vi "ESP Read-Write (SubVI) - C.vi"(0 "COM Port Input":refnum<visa-resource-name>, 5 "Command Input":T2, 7 "Manual Write Command":bool, 9 "Timeout (ms)":u32=10, 11 "Write/Read Wait (ms)":u32=10, 12 "Auto-Write on New Command?":bool=TRUE, 14 "Stop Program?":bool) -> (4 "ESP Values":T1, 15 "Error Output":errorcluster)   [LabVIEW 2011]
panel:
  # "ESP-D Read/Write (SubVI)\nCreated by Blake Otting - November 2009\nLast Updated - 2-29-2012"
  # "OUTPUTS"
  # "INPUTS"
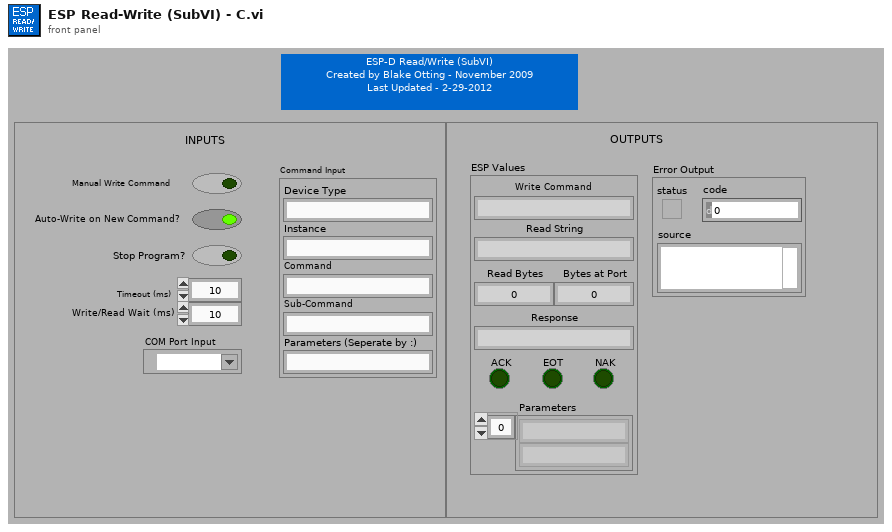
[diagram p1: front panel]
types:
  T1 = cluster{"Write Command":string, "Read String":string, "Read Bytes":u32, "Bytes at Port":u32, "Response":string, "ACK":bool, "EOT":bool, "NAK":bool, "Parameters":string[]}
  T2 = cluster{"Device Type":string, "Instance":string, "Command":string, "Sub-Command":string, "Parameters (Seperate by :)":string}
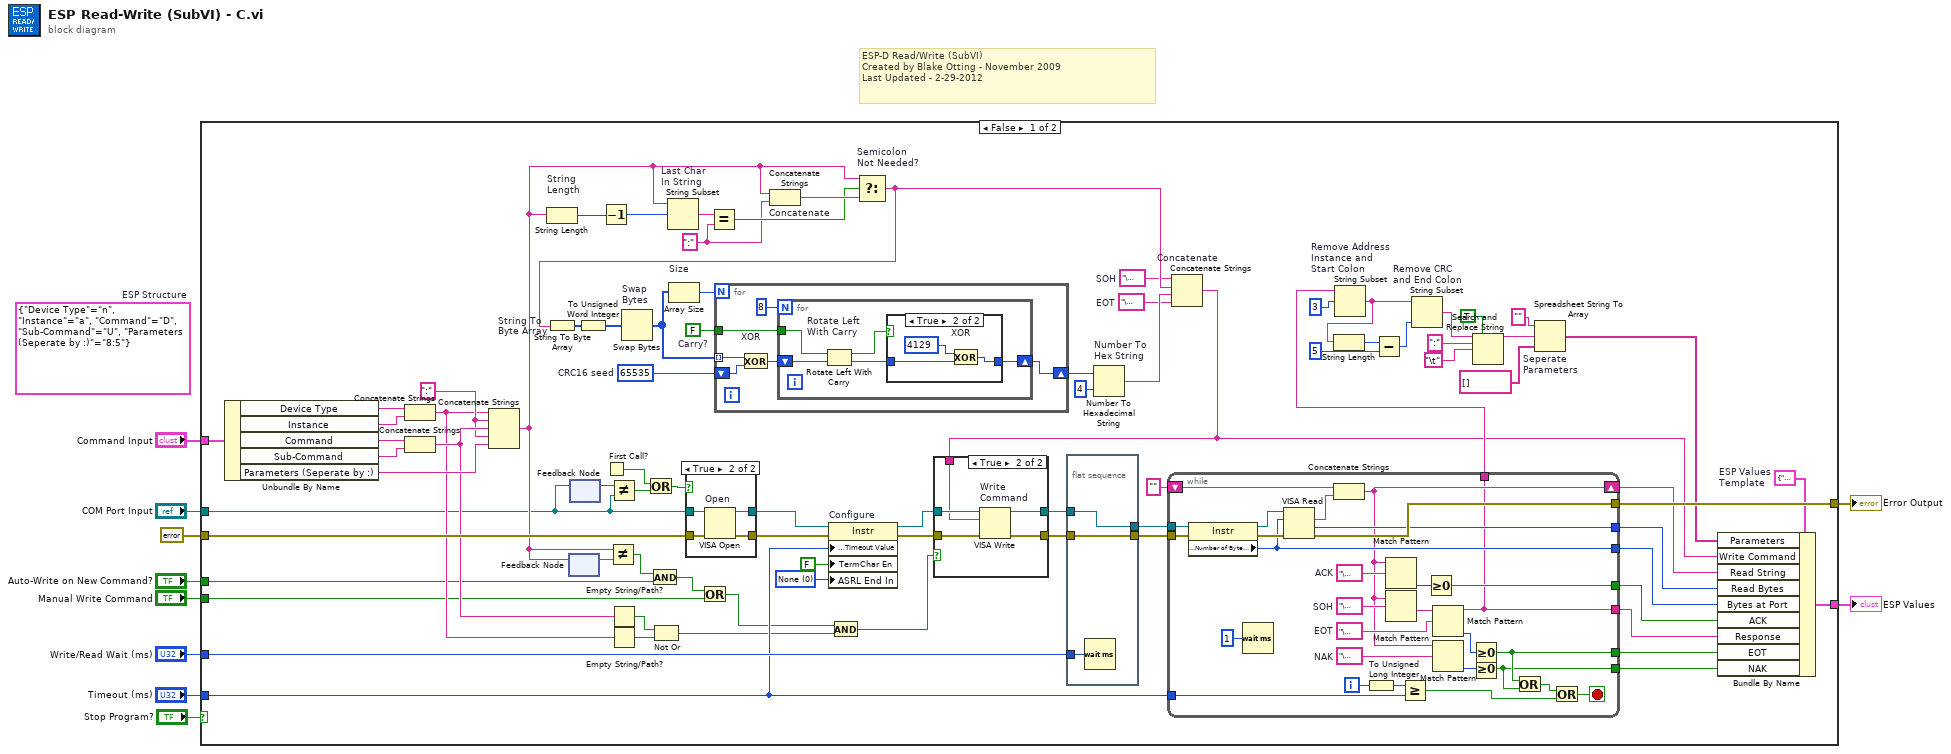
[diagram p0: block diagram]
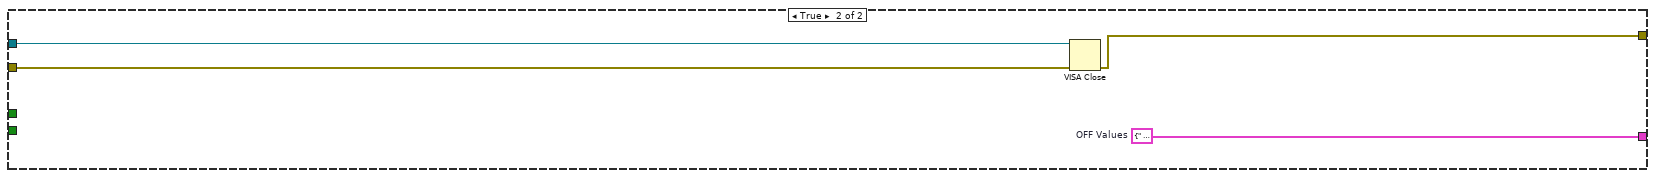
[diagram p5: hidden frame]
diagram:
  (unwired) T2 {"Device Type"="n", "Instance"="a", "Command"="D", "Sub-Command"="U", "Parameters (Seperate by :)"="8:5"}  # ESP Structure
  # "ESP-D Read/Write (SubVI)\nCreated by Blake Otting - November 2009\nLast Updated - 2-29-2012"
  n1 = case shown="False" "Stop Program?" {
    tunnel: "Auto-Write on New Command?" -> [w19 _]
    tunnel: "Command Input" -> [w92 _]
    tunnel: "Manual Write Command" -> [w18 _]
    tunnel: "Timeout (ms)" -> [w48 _]
    tunnel: "Write/Read Wait (ms)" -> [w91 _]
    tunnel: [w47 w154] -> w5
    tunnel: "COM Port Input" -> [w21 w156]
    tunnel: [w73 w153] -> w1
    tunnel: errorcluster {"status"=FALSE, "code"=0, "source"=""} ("error in (no error)") -> [w68 w155]
    frame False {
      w11 = FALSE  # Carry?
      w42 = T1 {"Write Command"="", "Read String"="", "Read Bytes"=0, "Bytes at Port"=0, "Response"="", "ACK"=FALSE, "EOT"=FALSE, "NAK"=FALSE, "Parameters"=[]}  # ESP Values  Template
      w49 = "\u0004"  # EOT
      w50 = "\u0001"  # SOH
      w85 = ":" ("y")
      w77 = u16 65535  # CRC16 seed
      w66 = u16 0 items=["None", "LastBit", "TermChar"] ("ASRLEndIn")
      w28 = ":"
      n2 = Unbundle By Name(w92) -> ("Device Type"=w34:string, "Instance"=w33:string, "Command"=w32:string, "Sub-Command"=w31:string, "Parameters (Seperate by :)"=w30:string)
      n3 = Concatenate Strings(w34, w33) -> (w27:string)
      n4 = Concatenate Strings(w32, w31) -> (w29:string)
      n5 = Concatenate Strings(w27, w28, w29, w28, w30) -> (w24:string)
      n6 = String Length "String\nLength"(string=w24) -> (length=w82:i32)
      n7 = feedback-in #1(w24) -> ()
      n8 = feedback #1() -> (w23:string)  [unwired: 1 in]
      n9 = feedback #2() -> (w22:refnum<visa-resource-name>)  [unwired: 1 in]
      n10 = feedback-in #2(w21) -> ()
      n11 = Decrement(x=w82) -> (x-1=w83:i32)
      n12 = First Call?() -> (First Call?: T/F=w13:bool)
      n13 = Not Equal?(x=w24, y=w23) -> (x != y?=w20:bool)
      n14 = Not Equal?(x=w22, y=w21) -> (x != y?=w12:bool)
      n15 = Empty String/Path?(string/path=w29) -> (empty?=w26:bool)
      n16 = Empty String/Path?(string/path=w27) -> (empty?=w25:bool)
      n17 = Or(x=w13, y=w12) -> (x .or. y?=w74:bool)
      n18 = And(x=w20, y=w19) -> (x .and. y?=w17:bool)
      n19 = Not Or(1:w25, 2:w26) -> (0:w15:bool)
      n20 = String Subset "Last Char\nIn String"(string=w24, offset (0)=w83) -> (substring=w84:string)  [unwired: 1 out]
      n21 = case shown="True" w74 {
        tunnel: w21 -> [w123 w127]
        tunnel: [w123 w126] -> w72
        tunnel: w68 -> [w122 w125]
        tunnel: [w122 w124] -> w71
        frame False {
        }
        frame True {
          n22 = VISA Open "Open"(error in (no error)=w125, VISA resource name=w127) -> (VISA resource name=w126:refnum<visa-resource-name>, error out=w124:errorcluster)  [unwired: 3 in]
        }
      }
      n23 = Or(x=w17, y=w18) -> (x .or. y?=w16:bool)
      n24 = Equal?(x=w84, y=w85) -> (x = y?=w86:bool)
      n25 = Concatenate Strings "Concatenate"(w24, w85) -> (w87:string)
      n26 = property on="Configure" class="Instr"(reference=w72, error in=w71, "General Settings:Timeout Value"=w48, "TermChar En"=FALSE ("enable"), "ASRL End In"=w66) -> (reference out=w70:refnum<visa-resource-name>, error out=w69:errorcluster)
      n27 = And(x=w16, y=w15) -> (x .and. y?=w14:bool)
      n28 = Select "Semicolon\nNot Needed?"(t=w24, s=w86, f=w87) -> (s? t:f=w88:string)
      n29 = String To Byte Array "String To \nByte Array"(string=w88) -> (unsigned byte array=w75:u8[])
      n30 = To Unsigned Word Integer ("To\nUNIT16")(number=w75) -> (unsigned 16bit integer=w76:u16[])
      n31 = Swap Bytes "Swap\nBytes"(anything=w76) -> (byte swapped=w79:u16[])
      n32 = Array Size "Size"(array=w79) -> (size(s)=w78:i32)
      n33 = for {
        N: w78 -> [_]
        shift-right: [w132] -> w80
        shift-left: w77 -> [w129]
        tunnel: w79 -> [w131] mode=indexing
        tunnel: w11 -> [w128]
        n34 = Exclusive Or "XOR"(1:w129, 2:w131) -> (0:w130:u16)
        n35 = for {
          N: 8 -> [_]
          shift-right: [w138] -> w132
          shift-left: w130 -> [w135]
          tunnel: w128 -> [w134]
          n36 = Rotate Left With Carry "Rotate Left\nWith Carry"(2:w135, 3:w134) -> (0:w136:u16, 1:w137:bool)
          n37 = case shown="True" w137 {
            tunnel: w136 -> [w139 w140]
            tunnel: [w139 w142] -> w138
            frame False {
            }
            frame True {
              n38 = Exclusive Or "XOR"(1:w140, 2:u16 4129) -> (0:w142:u16)
            }
          }
        }
      }
      n39 = flat-sequence {
        tunnel: w89 -> [w145]
        tunnel: [w145] -> w51
        tunnel: w90 -> [w144]
        tunnel: [w144] -> w52
        tunnel: w91 -> [w143]
        frame #0 {
          n40 = Wait (ms)(milliseconds to wait=w143) -> ()  [unwired: 1 out]
        }
      }
      n41 = Number To Hexadecimal String "Number To\nHex String"(1:i16 4 ("width (-)"), 2:w80) -> (0:w81:string)
      n42 = while {
        shift-left: "" -> [w120]
        shift-right: [w99] -> w43
        tunnel: w51 -> [w116]
        tunnel: w52 -> [w115]
        tunnel: [w117] -> w46
        tunnel: [w113] -> w45
        tunnel: w48 -> [w109]
        tunnel: [w94] -> w41
        tunnel: [w97] -> w44
        tunnel: [w96] -> w39
        tunnel: [w95] -> w38
        tunnel: [w118] -> w47
        tunnel: [w94] -> w40
        i -> [w108]
        stop <- w112 stop-if-true
        w101 = "\u0004"  # EOT
        w100 = "\u0001"  # SOH
        w104 = "\u0015"  # NAK
        w106 = "\u0006"  # ACK
        n43 = property class="Instr"(reference=w115, error in=w116) -> (reference out=w114:refnum<visa-resource-name>, error out=w121:errorcluster, "Serial Settings:Number of Bytes at Serial Port"=w113:u32)
        n44 = Wait (ms)(milliseconds to wait=u32 1) -> ()  [unwired: 1 out]
        n45 = VISA Read(VISA resource name=w114, byte count=w113, error in (no error)=w121) -> (read buffer=w119:string, return count=w117:u32, error out=w118:errorcluster)  [unwired: 1 out]
        n46 = Concatenate Strings(w120, w119) -> (w99:string)
        n47 = To Unsigned Long Integer(number=w108) -> (unsigned 32bit integer=w107:u32)
        n48 = Match Pattern(string=w99, regular expression=w106) -> (offset past match=w105:i32)  [unwired: 4 out]
        n49 = Match Pattern ("Find\nSOH")(string=w99, regular expression=w100) -> (after substring=w102:string)  [unwired: 4 out]
        n50 = Greater Or Equal?(x=w107, y=w109) -> (x >= y?=w111:bool)
        n51 = Greater Or Equal To 0?(x=w105) -> (x >= 0?=w97:bool)
        n52 = Match Pattern ("Find\nEOT")(string=w102, regular expression=w101) -> (before substring=w94:string, offset past match=w103:i32)  [unwired: 3 out]
        n53 = Match Pattern ("Find\nNAK")(string=w99, regular expression=w104) -> (offset past match=w98:i32)  [unwired: 4 out]
        n54 = Greater Or Equal To 0?(x=w103) -> (x >= 0?=w96:bool)
        n55 = Greater Or Equal To 0?(x=w98) -> (x >= 0?=w95:bool)
        n56 = Or(x=w96, y=w95) -> (x .or. y?=w110:bool)
        n57 = Or(x=w110, y=w111) -> (x .or. y?=w112:bool)
      }
      n58 = Concatenate Strings "Concatenate"(w50, w88, w81, w49) -> (w35:string)
      n59 = case shown="True" w14 {
        tunnel: [w147 w152] -> w90
        tunnel: w70 -> [w147 w151]
        tunnel: w69 -> [w146 w150]
        tunnel: [w146 w149] -> w89
        tunnel: w35 -> [_ w148]
        frame False {
        }
        frame True {
          n60 = VISA Write "Write\nCommand"(VISA resource name=w151, write buffer=w148, error in (no error)=w150) -> (VISA resource name out=w152:refnum<visa-resource-name>, error out=w149:errorcluster)  [unwired: 1 out]
        }
      }
      n61 = String Subset "Remove Address\nInstance and \nStart Colon"(string=w41, offset (0)=3) -> (substring=w60:string)  [unwired: 1 in]
      n62 = String Length(string=w60) -> (length=w64:i32)
      n63 = Subtract(x=w64, y=5) -> (x-y=w62:i32)
      n64 = String Subset "Remove CRC\nand End Colon"(string=w60, length (rest)=w62) -> (substring=w53:string)  [unwired: 1 in]
      n65 = Search and Replace String(replace all?=TRUE ("replace all? (F)"), input string=w53, search string=":", replace string="\t") -> (result string=w56:string)  [unwired: 4 in, 3 out]
      n66 = Spreadsheet String To Array "Seperate\nParameters"(format string="", spreadsheet string=w56, array type (2D Dbl)=string[] [] ("appended array")) -> (array=w37:string[])  [unwired: 1 in]
      n67 = Bundle By Name(cluster=w42, "Parameters"=w37, "Write Command"=w35, "Read String"=w43, "Read Bytes"=w46, "Bytes at Port"=w45, "ACK"=w44, "Response"=w40, "EOT"=w39, "NAK"=w38) -> (w73:T1)
    }
    frame True {
      w153 = T1 {"Write Command"=" ", "Read String"=" ", "Read Bytes"=0, "Bytes at Port"=0, "Response"=" ", "ACK"=FALSE, "EOT"=FALSE, "NAK"=FALSE, "Parameters"=["", "", "", " "]}  # OFF Values
      n68 = VISA Close(VISA resource name=w156, error in (no error)=w155) -> (error out=w154:errorcluster)
    }
  }
  "Error Output" <- w5
  "ESP Values" <- w1
